vi "LatchBool.vi"(7 "falling edge? (f)":bool, 11 "Boolean":bool) -> (3 "Latched Boolean":bool)   [LabVIEW 2019, in "RT_Game.lvlib" / "Engine.lvclass"]
uses:
  Engine.lvclass
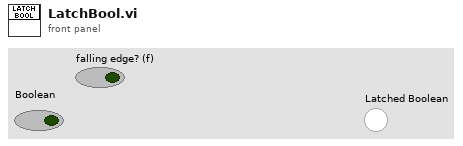
[diagram p1: front panel]
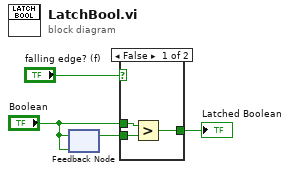
[diagram p0: block diagram]
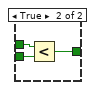
[diagram p2: hidden frame]
diagram:
  n1 = feedback-in #1("Boolean") -> ()
  n2 = feedback #1("Boolean") -> (w3:bool)
  n3 = case shown="False" "falling edge? (f)" {
    tunnel: "Boolean" -> [w7 w10]
    tunnel: w3 -> [w6 w9]
    tunnel: [w5 w8] -> w2
    frame False {
      n4 = Greater?(x=w7, y=w6) -> (0:w5:bool)
    }
    frame True {
      n5 = Less?(x=w10, y=w9) -> (x < y?=w8:bool)
    }
  }
  "Latched Boolean" <- w2
